vi "HW_6p1_Task1_PRADHASK.vi"() -> ()   [LabVIEW 2016]
uses:
  <vilib>/express/express arith-compare/Formula/XNode/ExpressFormulaBlockNode.xnode
panel:
  out "c":dbl
  in  "C":dbl
  in  "b":dbl
  in  "a":dbl
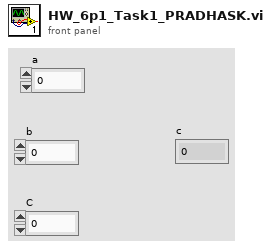
[diagram p1: front panel]
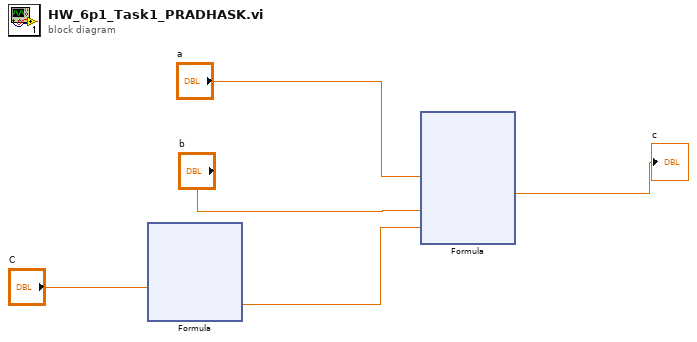
[diagram p0: block diagram]
diagram:
  n1 = xnode "Formula"("C"="C") -> ("Result"=w2:dbl)  [unwired: 1 in, 1 out]
  n2 = xnode "Formula"("a"="a", "b"="b", "C"=w2) -> ("Result"=→"c":dbl)  [unwired: 1 in, 1 out]
